vi "R1NH4SignalProcess.vi"(9 "error":errorcluster, 11 "LabVIEW Web Service":refnum<class "Web Service.lvclass">) -> (1 "error Out":errorcluster)   [LabVIEW 2016]
uses:
  <vilib>/wsapi/Web Service.lvclass
  Controls/ISE.ctl
  Controls/Tri State Control.ctl
panel:
  out "R1NH4":T1 {"Steady State?" items=["False", "True", "NaN", ""]}
  out "output array":dbl[][](array[numeric])
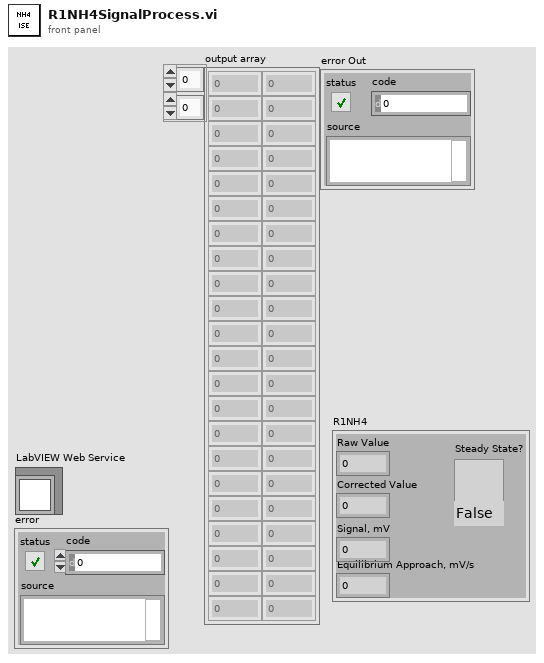
[diagram p1: front panel]
types:
  T1 = typedef "ISE.ctl" = cluster{"Raw Value":dbl, "Corrected Value":dbl, "Signal, mV":dbl, "Equilibrium Approach, mV/s":dbl, "Steady State?":T2}
  T2 = typedef "Tri State Control.ctl" = u16
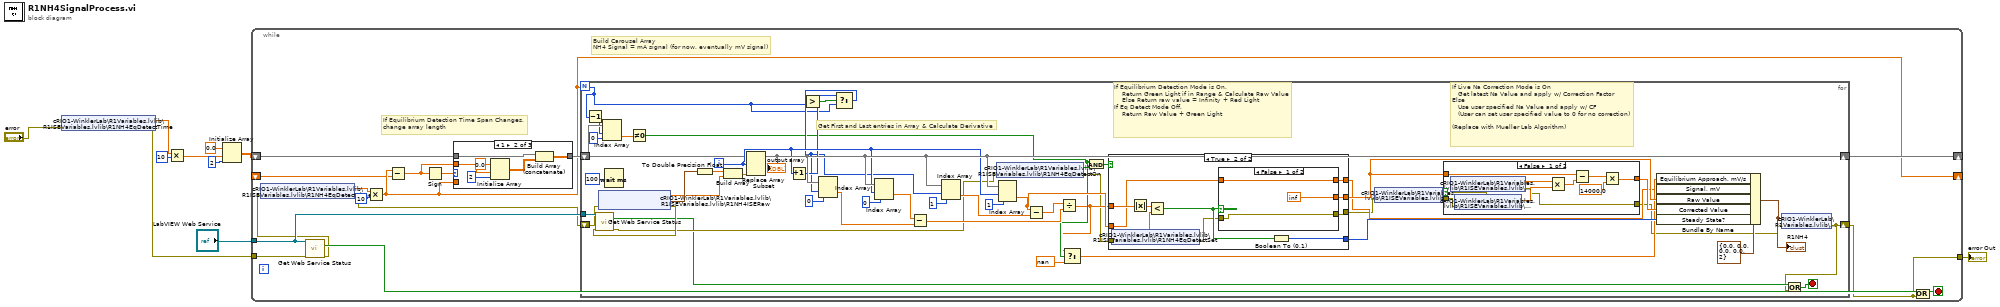
[diagram p0: block diagram]
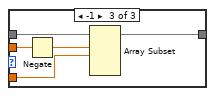
[diagram p3: hidden frame]
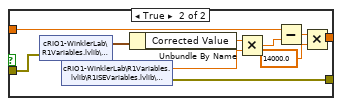
[diagram p4: hidden frame]
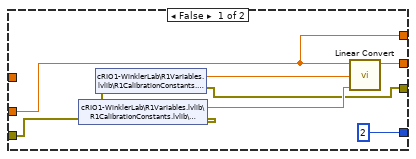
[diagram p5: hidden frame]
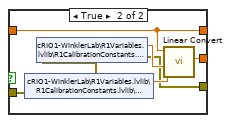
[diagram p6: hidden frame]
diagram:
  n1 = shared-variable "cRIO1-WinklerLab\\R1Variables.lvlib\\R1ISEVariables.lvlib\\R1NH4EqDetectTime"(error in="error") -> (w4:dbl, error out=w2:errorcluster)
  n2 = Multiply(x=w4, y=10) -> (x*y=w5:dbl)
  n3 = Initialize Array(0.0 ("element"), w5, 2 ("dimension size")) -> (w6:dbl[][])
  n4 = while {
    tunnel: "LabVIEW Web Service" -> [w26]
    tunnel: w2 -> [w15]
    shift-right: [w20] -> _
    shift-left: w6 -> [w23]
    shift-right: [w19] -> _
    shift-left: _ -> [w18]
    tunnel: [w11] -> w1
    stop <- w12 stop-if-true
    # "Build Carousel Array\nNH4 Signal = mA signal (for now, eventually mV signal)"
    # "If Equilibrium Detection Time Span Changes, \nchange array length"
    n5 = call <vilib>:"Get Web Service Status.vi"("LabVIEW Web Service"=w26, "error in (no error)"=w15) -> ("service stopping?"=w16:bool, "error out"=w14:errorcluster)  [unwired: 11 in, 1 out]
    n6 = shared-variable "cRIO1-WinklerLab\\R1Variables.lvlib\\R1ISEVariables.lvlib\\R1NH4EqDetectTime"(error in=w14) -> (w17:dbl, error out=w13:errorcluster)
    n7 = Multiply(x=w17, y=10) -> (x*y=w19:dbl)
    n8 = Subtract(x=w19, y=w18) -> (x-y=w22:dbl)
    n9 = Sign(1:w22) -> (0:w24:dbl)
    n10 = case shown="1" w24 {
      tunnel: w23 -> [w27 w31 w34]
      tunnel: w22 -> [_ w28 w36]
      tunnel: [w27 w29 w38] -> w21
      tunnel: w19 -> [_ _ w37]
      frame 0, Default {
      }
      frame 1 {
        n11 = Initialize Array(0.0 ("element"), w28, 2 ("dimension size")) -> (w30:dbl[][])
        n12 = Build Array (concatenate)(w31, w30) -> (w29:dbl[][])
      }
      frame -1 {
        n13 = Negate(x=w36) -> (-x=w35:dbl)
        n14 = Array Subset(array=w34, index (row)=w35, length (row)=w37) -> (w38:dbl[][])  [unwired: 2 in]
      }
    }
    n15 = for {
      N: w19 -> [w51]
      tunnel: w26 -> [w87]
      shift-right: [w73] -> w20
      shift-left: w21 -> [w63]
      shift-right: [w39] -> w11
      shift-left: w13 -> [w42]
      i -> [w72]
      stop <- w40 stop-if-true
      # "If Live Na Correction Mode is On\n   Get latest Na Value and apply w/ Correction Factor\nElse\n   Use user specified Na Value and apply w/ CF\n   (User can set user specified value to 0 for no correction)\n\n(Replace with Mueller Lab Algorithm)"
      # "If Equilibrium Detection Mode is On, \n    Return Green Light if in Range & Calculate Raw Value\n    Else Return raw value = Infinity + Red Light\nIf Eq Detect Mode Off,\n    Return Raw Value + Green Light"
      # "Get First and Last entries in Array & Calculate Derivative"
      n16 = Decrement(x=w51) -> (x-1=w52:i32)
      n17 = shared-variable "cRIO1-WinklerLab\\R1Variables.lvlib\\R1ISEVariables.lvlib\\R1NH4ISERaw"(error in=w42) -> (w69:dbl, error out=w48:errorcluster, w70:timestamp)
      n18 = call <vilib>:"Get Web Service Status.vi"("LabVIEW Web Service"=w87, "error in (no error)"=w48) -> ("service stopping?"=w41:bool, "error out"=w47:errorcluster)  [unwired: 11 in, 1 out]
      n19 = Index Array(array=w63, index (row)=w52, index (col)=0 ("disabled index (col)")) -> (element=w61:dbl)
      n20 = Wait (ms)(milliseconds to wait=u32 100) -> ()  [unwired: 1 out]
      n21 = Not Equal To 0?(x=w61) -> (x != 0?=w57:bool)
      n22 = To Double Precision Float(number=w70) -> (double precision float=w86:dbl)
      n23 = Build Array(w86, w69) -> (w85:dbl[])
      n24 = Replace Array Subset(array=w63, new element=w85, index (row)=w72) -> (w73:dbl[][])  [unwired: 1 in]
      "output array" <- w73
      n25 = Increment(x=w72) -> (x+1=w65:i32)
      n26 = Greater?(x=w65, y=w51) -> (0:w66:bool)
      n27 = Select(t=w65, s=w66, f=w51) -> (s? t:f=w64:i32)
      n28 = Index Array(array=w73, index (row)=w64, index (col)=0 ("disabled index (col)")) -> (element=w75:dbl)
      n29 = Index Array(array=w73, index (row)=w72, index (col)=0 ("disabled index (col)")) -> (element=w68:dbl)
      n30 = Subtract(x=w68, y=w75) -> (x-y=w81:dbl)
      n31 = Index Array(array=w73, index (row)=w64, index (col)=1 ("disabled index (col)")) -> (element=w74:dbl)
      n32 = shared-variable "cRIO1-WinklerLab\\R1Variables.lvlib\\R1ISEVariables.lvlib\\R1NH4EqDetectOn"(error in=w47) -> (w60:bool, error out=w46:errorcluster)
      n33 = Index Array(array=w73, index (row)=w72, index (col)=1 ("disabled index (col)")) -> (element=w58:dbl)
      n34 = Subtract(x=w58, y=w74) -> (x-y=w80:dbl)
      n35 = Divide(x=w80, y=w81) -> (x/y=w55:dbl)
      n36 = Select(t=w55, s=w57, f=nan) -> (s? t:f=w54:dbl)
      n37 = And(x=w57, y=w60) -> (x .and. y?=w59:bool)
      n38 = case shown="True" w59 {
        tunnel: [w112 w127] -> w82
        tunnel: [w115 w126] -> w53
        tunnel: w55 -> [_ w125]
        tunnel: [2 w123] -> w71
        tunnel: w58 -> [w115 w122]
        tunnel: w46 -> [w111 w119]
        tunnel: [w109 w117] -> w45
        frame False {
          n39 = shared-variable "cRIO1-WinklerLab\\R1Variables.lvlib\\R1CalibrationConstants.lvlib\\R1NH4Intercept"(error in=w111) -> (w114:dbl, error out=w110:errorcluster)
          n40 = shared-variable "cRIO1-WinklerLab\\R1Variables.lvlib\\R1CalibrationConstants.lvlib\\R1NH4Slope"(error in=w110) -> (w113:dbl, error out=w109:errorcluster)
          n41 = call "Linear Convert.vi"("Intercept"=w114, "Slope"=w113, "Signal"=w115) -> ("Result"=w112:dbl)  [unwired: 8 in]
        }
        frame True {
          n42 = shared-variable "cRIO1-WinklerLab\\R1Variables.lvlib\\R1ISEVariables.lvlib\\R1NH4EqDetectSet"(error in=w119) -> (w121:dbl, error out=w118:errorcluster)
          n43 = Absolute Value(x=w125) -> (abs(x)=w120:dbl)
          n44 = Less?(x=w120, y=w121) -> (x < y?=w124:bool)
          n45 = case shown="False" w124 {
            tunnel: [inf w136] -> w127
            tunnel: [w129 w137] -> w126
            tunnel: w122 -> [w129 w137]
            tunnel: w118 -> [w128 w133]
            tunnel: [w128 w131] -> w117
            frame False {
            }
            frame True {
              n46 = shared-variable "cRIO1-WinklerLab\\R1Variables.lvlib\\R1CalibrationConstants.lvlib\\R1NH4Intercept"(error in=w133) -> (w135:dbl, error out=w132:errorcluster)
              n47 = shared-variable "cRIO1-WinklerLab\\R1Variables.lvlib\\R1CalibrationConstants.lvlib\\R1NH4Slope"(error in=w132) -> (w134:dbl, error out=w131:errorcluster)
              n48 = call "Linear Convert.vi"("Intercept"=w135, "Slope"=w134, "Signal"=w137) -> ("Result"=w136:dbl)  [unwired: 8 in]
            }
          }
          n49 = Boolean To (0,1)(Boolean=w124) -> (0, 1=w123:i16)
        }
      }
      n50 = shared-variable "cRIO1-WinklerLab\\R1Variables.lvlib\\R1ISEVariables.lvlib\\R1NH4NaOn"(error in=w45) -> (w67:bool, error out=w44:errorcluster)
      n51 = case shown="False" w67 {
        tunnel: w82 -> [w94 w106]
        tunnel: [w93 w103] -> w83
        tunnel: w44 -> [w90 w100]
        tunnel: [w88 w98] -> w43
        frame False {
          n52 = shared-variable "cRIO1-WinklerLab\\R1Variables.lvlib\\R1ISEVariables.lvlib\\R1NH4NaCF"(error in=w90) -> (w92:dbl, error out=w89:errorcluster)
          n53 = shared-variable "cRIO1-WinklerLab\\R1Variables.lvlib\\R1ISEVariables.lvlib\\R1NH4NaConc"(error in=w89) -> (w91:dbl, error out=w88:errorcluster)
          n54 = Multiply(x=w91, y=w92) -> (x*y=w95:dbl)
          n55 = Subtract(x=w94, y=w95) -> (x-y=w97:dbl)
          n56 = Multiply(x=w97, y=14000.0) -> (x*y=w93:dbl)
        }
        frame True {
          n57 = shared-variable "cRIO1-WinklerLab\\R1Variables.lvlib\\R1Signals.lvlib\\R1Na"(error in=w100) -> (w101:T1, error out=w99:errorcluster)
          n58 = shared-variable "cRIO1-WinklerLab\\R1Variables.lvlib\\R1ISEVariables.lvlib\\R1NH4NaCF"(error in=w99) -> (w102:dbl, error out=w98:errorcluster)
          n59 = Unbundle By Name(w101) -> ("Corrected Value"=w107:dbl)
          n60 = Multiply(x=w107, y=w102) -> (x*y=w108:dbl)
          n61 = Subtract(x=w106, y=w108) -> (x-y=w104:dbl)
          n62 = Multiply(x=w104, y=14000.0) -> (x*y=w103:dbl)
        }
      }
      n63 = Bundle By Name(cluster=T1 {"Raw Value"=0.0, "Corrected Value"=0.0, "Signal, mV"=0.0, "Equilibrium Approach, mV/s"=0.0, "Steady State?"=2} ("R1NH4"), "Equilibrium Approach, mV/s"=w54, "Signal, mV"=w53, "Raw Value"=w82, "Corrected Value"=w83, "Steady State?"=w71) -> (w49:T1)
      "R1NH4" <- w49
      n64 = shared-variable "cRIO1-WinklerLab\\R1Variables.lvlib\\R1Signals.lvlib\\R1NH4"(w49, error in=w43) -> (error out=w39:errorcluster)
      n65 = Or(x=w41, y=w39) -> (x .or. y?=w40:bool)
    }
    n66 = Or(x=w16, y=w11) -> (x .or. y?=w12:bool)
  }
  "error Out" <- w1
